vi "ExtractModuleID.vi"(7 "ModuleType":string="AcPwr", 8 "error in":errorcluster, 10 "Parameter List":variant, 11 "Test.lvclass In":refnum<class "Test.lvclass">) -> (0 "Error Out":errorcluster, 1 "ModuleIDs":i32, 2 "ErrorSeverity":string, 3 "Test.lvclass Out":refnum<class "Test.lvclass">, 4 "Variant Output(Module List for Debugging)":variant, 6 "Parameter List":string[](array[string]))   [LabVIEW 2018, in "Test.lvclass"]
doc: "Parses the incoming message variant and determines if the message should be sent to all clones ( specific to a given module) or a specific clone in that module."
uses:
  Test.lvclass
  Test.lvclass/Test.ctl
  Accessors/Read ErrorSeverity.vi
  Accessors/Read ModuleIDs.vi
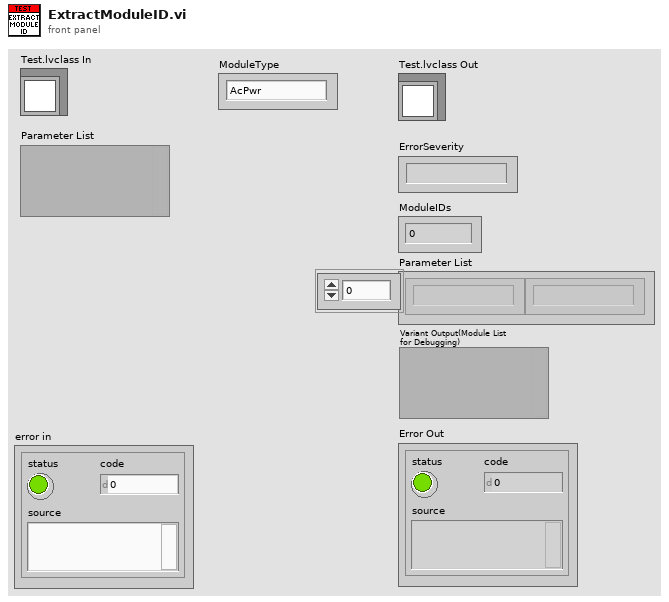
[diagram p1: front panel]
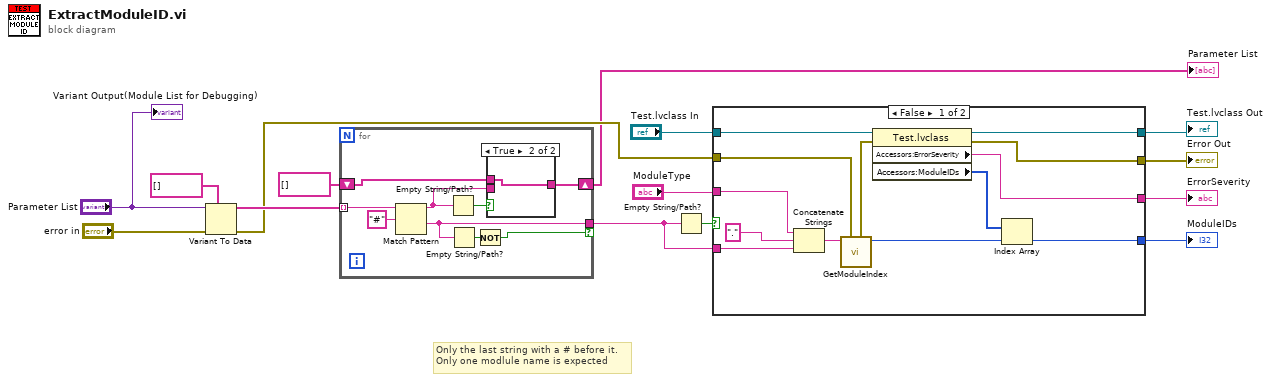
[diagram p0: block diagram]
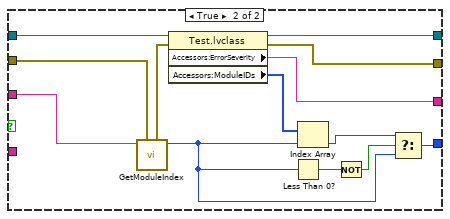
[diagram p2: hidden frame]
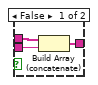
[diagram p3: hidden frame]
diagram:
  # "Only the last string with a # before it.\nOnly one modlule name is expected"
  n1 = Variant To Data(error in="error in", type=string[] [], Variant="Parameter List") -> (data=w15:string[], error out=w13:errorcluster)
  n2 = for {
    tunnel: w15 -> [w24] mode=indexing
    tunnel: [w18] -> w14 if=w16
    shift-right: [w20] -> w5
    shift-left: string[] [] -> [w19]
    n3 = Match Pattern(string=w24, regular expression="#") -> (before substring=w21:string, after substring=w18:string)  [unwired: 1 in, 2 out]
    n4 = Empty String/Path?(string/path=w21) -> (empty?=w22:bool)
    n5 = Empty String/Path?(string/path=w18) -> (empty?=w17:bool)
    n6 = Not(x=w17) -> (.not. x?=w16:bool)
    n7 = case shown="True" w22 {
      tunnel: w21 -> [w27 _]
      tunnel: [w26 w28] -> w20
      tunnel: w19 -> [w25 w28]
      frame False {
        n8 = Build Array (concatenate)(w25, w27) -> (w26:string[])
      }
      frame True {
      }
    }
  }
  "Parameter List" <- w5
  n9 = Empty String/Path?(string/path=w14) -> (empty?=w6:bool)
  n10 = case shown="False" w6 {
    tunnel: w13 -> [w41 w54]
    tunnel: w14 -> [w38 _]
    tunnel: "Test.lvclass In" -> [w36 w52]
    tunnel: [w35 w51] -> w10
    tunnel: [w34 w50] -> w9
    tunnel: [w31 w46] -> w8
    tunnel: [w32 w48] -> w7
    tunnel: "ModuleType" -> [w29 w47]
    frame False {
      n11 = Concatenate Strings(w29, "." ("string"), w38) -> (w39:string)
      n12 = call "GetModuleIndex.vi"("Error In"=w41, "ModuleType"=w39) -> ("ModuleIndex"=w30:i32, "Error"=w33:errorcluster)  [unwired: 8 in]
      n13 = property class="Test.lvclass"(reference=w36, error in=w33) -> (reference out=w35:refnum<class "Test.lvclass">, error out=w34:errorcluster, "Accessors:ErrorSeverity"=w32:string, "Accessors:ModuleIDs"=w37:i32[])
      n14 = Index Array(array=w37, index=w30) -> (element=w31:i32)
    }
    frame True {
      n15 = call "GetModuleIndex.vi"("Error In"=w54, "ModuleType"=w47) -> ("ModuleIndex"=w42:i32, "Error"=w49:errorcluster)  [unwired: 8 in]
      n16 = property class="Test.lvclass"(reference=w52, error in=w49) -> (reference out=w51:refnum<class "Test.lvclass">, error out=w50:errorcluster, "Accessors:ErrorSeverity"=w48:string, "Accessors:ModuleIDs"=w53:i32[])
      n17 = Less Than 0?(x=w42) -> (x < 0?=w44:bool)
      n18 = Index Array(array=w53, index=w42) -> (element=w45:i32)
      n19 = Not(x=w44) -> (.not. x?=w43:bool)
      n20 = Select(t=w45, s=w43, f=w42) -> (s? t:f=w46:i32)
    }
  }
  "Error Out" <- w9
  "ModuleIDs" <- w8
  "Test.lvclass Out" <- w10
  "ErrorSeverity" <- w7
  "Variant Output(Module List for Debugging)" <- "Parameter List"
